vi "niHWS Write Digital U8.vi"(8 "error in (no error)":errorcluster, 10 "data":u8[](array[numeric]), 11 "waveform reference in":u32) -> (0 "error out":errorcluster, 3 "waveform reference out":u32)   [LabVIEW 2020]
doc: "Writes an array of 8-bit unsigned integer (U8) digital waveform data into the file beginning at the current read/write position."
uses:
  nihwsu.dll
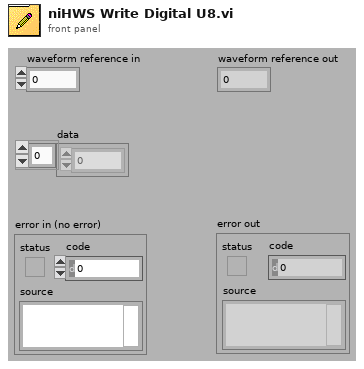
[diagram p1: front panel]
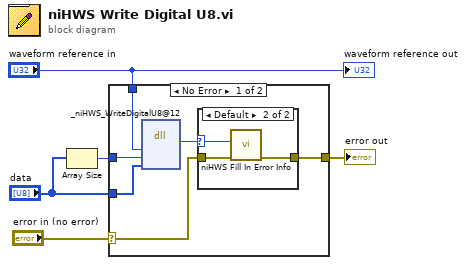
[diagram p0: block diagram]
diagram:
  n1 = Array Size(array="data") -> (size(s)=w1:i32)
  n2 = case shown="No Error" "error in (no error)" {
    selector: "error in (no error)" -> [w9 w16]
    tunnel: [w10 w16] -> w4
    tunnel: "waveform reference in" -> [w11 _]
    tunnel: "data" -> [w7 _]
    tunnel: w1 -> [w6 _]
    frame No Error {
      n3 = dll-call lib="nihwsu.dll" fn="_niHWS_WriteDigitalU8@12"("wfmReference"=w11, "numSamples"=w6, "wfmData"=w7) -> (w8:i32)  [unwired: 6 in, 2 out]
      n4 = case shown="Default" w8 {
        selector: w8 -> [_ w13]
        tunnel: [w12 w14] -> w10
        tunnel: w9 -> [w12 w15]
        frame 0 {
        }
        frame Default {
          n5 = call "niHWS Fill In Error Info.vi"("error in (no error)"=w15, "status code"=w13) -> ("error out"=w14:errorcluster)  [unwired: 9 in]
        }
      }
    }
    frame Error {
    }
  }
  "error out" <- w4
  "waveform reference out" <- "waveform reference in"
